vi "Enable Gain Ranging.vi"(0 "session in":T1[](array[typedef]) {"rx baseband session"."3630 session"."Address Space" items=["VXI/VME A16"=1, "VXI/VME A24"=2, "VXI/VME A32"=3, "VXI/VME A64"=4, "PXI Memory Allocations"=9, "PXI Configuration"=10, "PXI BAR0"=11, "PXI BAR1"=12, "PXI BAR2"=13, "PXI BAR3"=14, "PXI BAR4"=15, "PXI BAR5"=16]; "tx baseband session"."3610 session"."Address Space" items=["VXI/VME A16"=1, "VXI/VME A24"=2, "VXI/VME A32"=3, "VXI/VME A64"=4, "PXI Memory Allocations"=9, "PXI Configuration"=10, "PXI BAR0"=11, "PXI BAR1"=12, "PXI BAR2"=13, "PXI BAR3"=14, "PXI BAR4"=15, "PXI BAR5"=16]}, 1 "scope":string(combo), 5 "enable":bool=TRUE, 7 "TRx LO auto-muting":bool=TRUE, 11 "error in":errorcluster) -> (4 "session out":T1[](array[typedef]) {"rx baseband session"."3630 session"."Address Space" items=["VXI/VME A16"=1, "VXI/VME A24"=2, "VXI/VME A32"=3, "VXI/VME A64"=4, "PXI Memory Allocations"=9, "PXI Configuration"=10, "PXI BAR0"=11, "PXI BAR1"=12, "PXI BAR2"=13, "PXI BAR3"=14, "PXI BAR4"=15, "PXI BAR5"=16]; "tx baseband session"."3610 session"."Address Space" items=["VXI/VME A16"=1, "VXI/VME A24"=2, "VXI/VME A32"=3, "VXI/VME A64"=4, "PXI Memory Allocations"=9, "PXI Configuration"=10, "PXI BAR0"=11, "PXI BAR1"=12, "PXI BAR2"=13, "PXI BAR3"=14, "PXI BAR4"=15, "PXI BAR5"=16]}, 15 "error out":errorcluster)   [LabVIEW 2019]
uses:
  TypeDefs/Session.ctl
  <instrlib>/niMmWave/ni3620/Config/v1/Host/Public/High-Level/niMmWave Session.ctl
  <instrlib>/_niInstr/Register Bus/v0/Host/Public/Register Bus Session.ctl
  <instrlib>/_niInstr/Register Bus/v0/Host/Private/Session Data.ctl
  <instrlib>/niMmWave/ni3620/Config/v1/Host/Public/Typedefs/Board Information.ctl
  <instrlib>/niMmWave/ni3620/Config/v1/Host/Public/Typedefs/Hardware Revision.ctl
  <instrlib>/niMmWave/ni3620/Config/v1/Host/Public/Typedefs/Gain Mapping.ctl
  <instrlib>/niMmWave/ni3620/Config/v1/Host/Public/Typedefs/Correction Data.ctl
  <instrlib>/niMmWave/ni3620/Config/v1/Host/Public/Typedefs/Opera Characterization.ctl
  <instrlib>/niMmWave/ni3620/Config/v1/Host/Public/Corrections/Typedefs/Opera Characterization Main Header.ctl
  <instrlib>/niMmWave/ni3620/Config/v1/Host/Public/Corrections/Typedefs/Opera IF Board Information.ctl
  <instrlib>/niMmWave/ni3620/Config/v1/Host/Public/Corrections/Typedefs/Opera Characterization Instance Header.ctl
  <instrlib>/niMmWave/ni3620/Config/v1/Host/Public/Corrections/Typedefs/Opera Characterization Device Data Header.ctl
  <instrlib>/niMmWave/ni3620/Config/v1/Host/Public/Corrections/Typedefs/Opera LO Characterization Data Header.ctl
  <instrlib>/niMmWave/ni3620/Config/v1/Host/Public/Corrections/Typedefs/Opera IF Board Characterization Data Header.ctl
  <instrlib>/niMmWave/ni3620/Config/v1/Host/Public/Corrections/Typedefs/Opera Characterization Device Data.ctl
  <instrlib>/niMmWave/ni3620/Config/v1/Host/Public/Corrections/Typedefs/Opera LO2 Board Characterization Data.ctl
  <instrlib>/niMmWave/ni3620/Config/v1/Host/Public/Corrections/Typedefs/Opera LO Characterization Data.ctl
  <instrlib>/niMmWave/ni3620/Config/v1/Host/Public/Corrections/Typedefs/Opera IF Board Characterization Data.ctl
  <instrlib>/niMmWave/ni3620/Config/v1/Host/Public/Corrections/Typedefs/Opera IQ Impairment Data.ctl
  <instrlib>/niMmWave/ni3620/Config/v1/Host/Public/Typedefs/mmWave Adapter Session Data.ctl
  <instrlib>/niMmWave/ni3620/Config/v1/Host/Public/Typedefs/mmWave Adapter Data.ctl
  <instrlib>/niMmWave/ni3620/Config/v1/Host/Public/Typedefs/mmWave Adapter 2.ctl
  <instrlib>/niMmWave/ni3620/Config/v1/Shared/Typedefs/Subsystem ID.ctl
  <instrlib>/niMmWave/ni3620/Config/v1/Host/Public/Typedefs/mmWave Adapter Channel Information.ctl
  <instrlib>/niMmWave/ni3620/Config/v1/Host/Public/Typedefs/Temperature Coefficients.ctl
  <instrlib>/niMmWave/ni3620/Config/v1/Host/Public/Typedefs/mmWave Characterization.ctl
  <instrlib>/niMmWave/ni3620/Config/v1/Host/Public/Corrections/Typedefs/mmWave Characterization Main Header.ctl
  <instrlib>/niMmWave/ni3620/Config/v1/Host/Public/Corrections/Typedefs/mmWave Characterization Instance Header.ctl
  <instrlib>/niMmWave/ni3620/Config/v1/Host/Public/Typedefs/Session Cache.ctl
  <instrlib>/niMmWave/ni3620/Config/v1/Host/Public/Typedefs/LO2 settings cache.ctl
  <instrlib>/niMmWave/ni3620/Config/v1/Host/Public/Typedefs/LO2 source.ctl
  <instrlib>/niMmWave/ni3620/Config/v1/Host/Public/Typedefs/Desired and Coerced.ctl
  <instrlib>/niMmWave/ni3620/Config/v1/Host/Public/Typedefs/Export cache.ctl
  <instrlib>/niMmWave/ni3620/Config/v1/Host/Public/Typedefs/Path cache.ctl
  <instrlib>/niMmWave/ni3620/Config/v1/Host/Public/Typedefs/Daughterboard Type.ctl
  <instrlib>/niMmWave/ni3620/Config/v1/Host/Public/Typedefs/LO1 settings cache.ctl
  <instrlib>/niMmWave/ni3620/Config/v1/Host/Public/Typedefs/LO1 Source.ctl
  <instrlib>/niMmWave/ni3620/Config/v1/Host/Public/Typedefs/mmWave export cache.ctl
  <instrlib>/niMmWave/ni3620/Config/v1/Host/Private/Board/LO2/LO2 Board Configuration Cache.ctl
  <instrlib>/niMmWave/ni3620/Config/v1/Host/Public/Typedefs/reference clock routing settings.ctl
  <instrlib>/niMmWave/ni3620/Config/v1/Host/Public/Typedefs/LO2 routing settings.ctl
  <instrlib>/niMmWave/ni3620/Config/v1/Host/Private/Board/LO1/LO1 Board Configuration Cache.ctl
  <instrlib>/niMmWave/ni3620/Config/v1/Host/Public/Typedefs/LO1 source settings.ctl
  <instrlib>/niMmWave/ni3620/Config/v1/Host/Public/Typedefs/LO1 export settings.ctl
  <instrlib>/niMmWave/ni3620/Config/v1/Host/Public/Typedefs/LO1 mmWave settings.ctl
  TypeDefs/Tx Baseband Session.ctl
  <instrlib>/niMmWave/ni3610 and ni3630/controls/public/Main Settings.ctl
  <vilib>/Instr/_visa.llb/VISA Register Access Address Space.ctl
  <instrlib>/niMmWave/ni3610 and ni3630/controls/public/Register Adresses.ctl
  <instrlib>/niMmWave/ni3610 and ni3630/controls/public/Base Card Type.ctl
  <instrlib>/niMmWave/ni3610 and ni3630/controls/private/IQ Card Revision.ctl
  <instrlib>/niMmWave/ni3610 and ni3630/controls/public/Board Capability.ctl
  TypeDefs/Blank FPGA Reference.ctl
  TypeDefs/Rx Baseband Session.ctl
  TypeDefs/Hardware Configuration.ctl
  TypeDefs/Direction.ctl
  TypeDefs/Gain Ranging.ctl
  TypeDefs/PXI Trigger Bus Info.ctl
  TypeDefs/Gain Ranging Reference.ctl
  <vilib>/rvi/errors/niLvFpgaAdjustHostInterfaceError.vi
  <vilib>/FPGAPlugInAG/Dynamic/niLvFpga_P2PGetEndpoint_Dynamic.vi
  <vilib>/rvi/interface/nirviReadWriteControl/nirviReadWriteControl.xnode
  <vilib>/rvi/interface/nirviMethod/nirviMethod.xnode
  <instrlib>/niMmWave/ni3620/Config/v1/Host/niMmWave Config v1 Host.lvlib
  <vilib>/rvi/interface/Simulation/niFpgaSimulationCallBeginRW.vi
  NiFpgaLv.dll
  <vilib>/rvi/errors/niLvFpgaMergeErrorWithErrorCode.vi
  <instrlib>/_niInstr/Register Bus/v0/Host/niInstr Register Bus v0 Host.lvlib
  <instrlib>/niMmWave/ni3610 and ni3630/ni3610_and_ni3630_Driver_Lib.lvlib
  <instrlib>/niMmWave/ni3620/Config/v1/Shared/niMmWave Config v1 Shared.lvlib
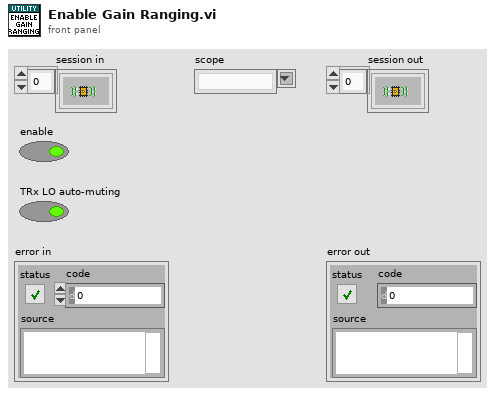
[diagram p1: front panel]
types:
  T1 = typedef "Session.ctl" = cluster{"3620 session":refnum<queue>, "tx baseband session":T2, "rx baseband session":T10, "tx gain (dB)":dbl, "rx gain (dB)":dbl, "hardware configuration":T11, "gain ranging":T13[], "pxi trigger bus information":T14}
  T2 = typedef "Tx Baseband Session.ctl" = cluster{"3610 session":T3, "7902 reference":T9}
  T3 = typedef "ni3610_and_ni3630_Driver_Lib.lvlib/Main Settings.ctl" = cluster{"VISA resource name":refnum<visa-resource-name>, "Address Space":T4, "window_offset":u32, "register_addresses":T5, "required_MM_fpga_version":cluster{"signature":u32, "hardware":u32, "current revision":u32, "oldest revision":u32}, "CPLD Oldest Compat Version ":cluster{"hardware":u32, "CPLD firmware":u32}, "MM_FPGA_image_location":string, "is_init":bool, "card_type":T6, "DacLmkConfigFileName":string, "AdcLmkConfigFileName":string, "AdcConfigFileName":string, "DacConfigFileName_RevA":string, "DacConfigFileName_RevB":string, "Mulde hardware revision":u8, "bypass DAC PLL\n":bool, "IQ Card Revision":T7, "board capability":T8}
  T4 = typedef "VISA Register Access Address Space.ctl" = u16
  T5 = typedef "ni3610_and_ni3630_Driver_Lib.lvlib/Register Adresses.ctl" = cluster{"MM based Registers":cluster{"Revision":u32, "OldestCompatRev":u32, "signature":u32, "scratch":u32, "LedControl":u32, "BoardHwRev":u32, "BoardControl":u32, "ThermalStatus":u32, "BasebandStatus":u32, "BasebandControl":u32, "BasebandAuxSetup":u32, "BasebandAuxStatus":u32, "LmkSyncOutSetup":u32, " AdcSyncOutSetup":u32, " InjSyncOutSetup":u32, " PxiTrig0OutSetup":u32, " PxiTrig1OutSetup":u32, " PxiTrig2OutSetup":u32, " PxiTrig3OutSetup":u32, " PxiTrig4OutSetup":u32, " PxiTrig5OutSetup":u32, " PxiTrig6OutSetup":u32, " PxiTrig7OutSetup":u32}, "CPLD based Registers":cluster{"SlaveSignature":u32, "SlaveRevision":u32, "SlaveOldestCompatRev":u32, "SlaveScratch":u32, "SlaveSetup":u32, "SlaveStatus":u32, "IDacReg_offset":u32, "LMKRegGrp0_offset":u32, "QDacReg_offset":u32, "BrdTempSensorVal":u32, "TempSensorPowerDown":u32, "GPIOReg_offset":u32, "IAdcReg_offset":u32, "QAdcReg_offset":u32, "LMKRegGrp1_offset":u32, "QadcTempSensorVal":u32, "IadcTempSensorVal":u32, "RevisionReg":u32, "VcxoReg":u32, "CpldStatusReg":u32, "PowerReg":u32, "VBiasEnReg":u32, "ExtRefOeReg":u32, "QdacCtrlReg":u32, "QdacStatusReg":u32, "IdacCtrlReg":u32, "IdacStatusReg":u32, "QdacJtagIn":u32, "QdacJtagOut":u32, "IdacJtagIn":u32, "IdacJtagOut":u32, "IqDcSetupReg":u32, "QadcStatusReg":u32, "IadcStatusReg":u32, "BrdSetupReg":u32, "IqDcRevisionReg":u32, "PllStatusReg":u32, "EndpointScratchReg":u32, "AdcSyncCfgReg":u32, "IqCardOpampReg":u32}, "CPLD Register Offset":u32, "MM  Register Offset":u32, " PxiTrig0OutSetup":u32}
  T6 = typedef "ni3610_and_ni3630_Driver_Lib.lvlib/Base Card Type.ctl" = enum16{"unspecified", "ADC", "DAC"}
  T7 = typedef "ni3610_and_ni3630_Driver_Lib.lvlib/IQ Card Revision.ctl" = enum16{"RevA", "RevB", "RevC", "RevD"}
  T8 = typedef "ni3610_and_ni3630_Driver_Lib.lvlib/Board Capability.ctl" = cluster{"baseband sync":enum16{"no baseband sync", "baseband sync"}}
  T9 = typedef "Blank FPGA Reference.ctl" = refnum<k20>
  T10 = typedef "Rx Baseband Session.ctl" = cluster{"3630 session":T3, "7902 reference":T9}
  T11 = typedef "Hardware Configuration.ctl" = cluster{"direction":T12, "baseband only":bool}
  T12 = typedef "Direction.ctl" = enum16{"Transceiver", "Receiver", "Transmitter"}
  T13 = typedef "Gain Ranging.ctl" = cluster{"gain ranging active scope":string, "gain ranging stream session":refnum<k20>}
  T14 = typedef "PXI Trigger Bus Info.ctl" = cluster{"chassis resource name":refnum<visa-resource-name>, "7902R (TX)":i16, "3610 (TX)":i16, "3620 (IF)":i16, "3630 (RX)":i16, "7902R (RX)":i16}
  T15 = typedef "Gain Ranging Reference.ctl" = refnum<k20>
  T16 = cluster{"shift step":i16, "base gain":fxp<+/-,16,12>}
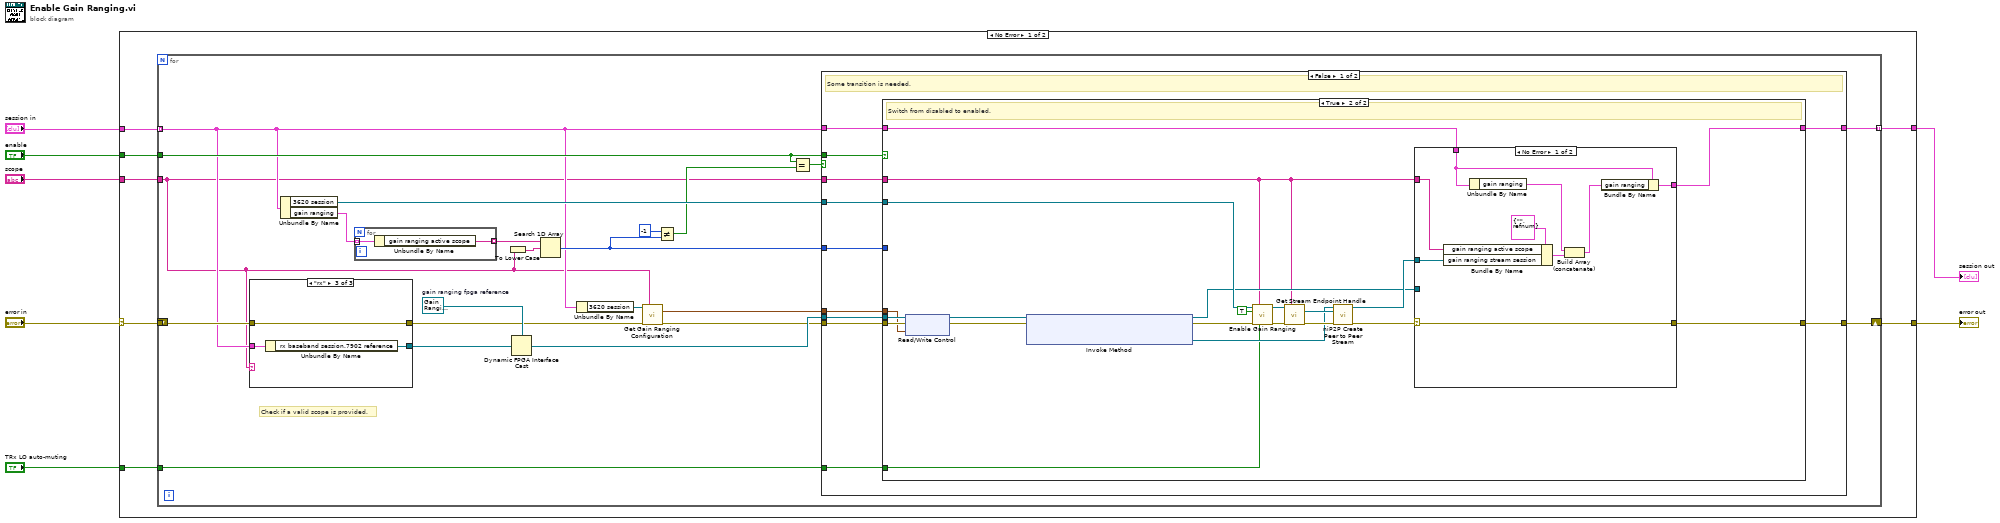
[diagram p0: block diagram]
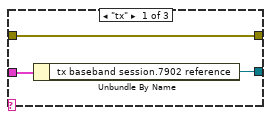
[diagram p2: hidden frame]
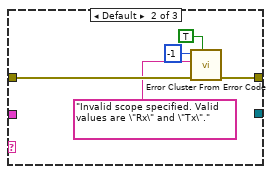
[diagram p3: hidden frame]
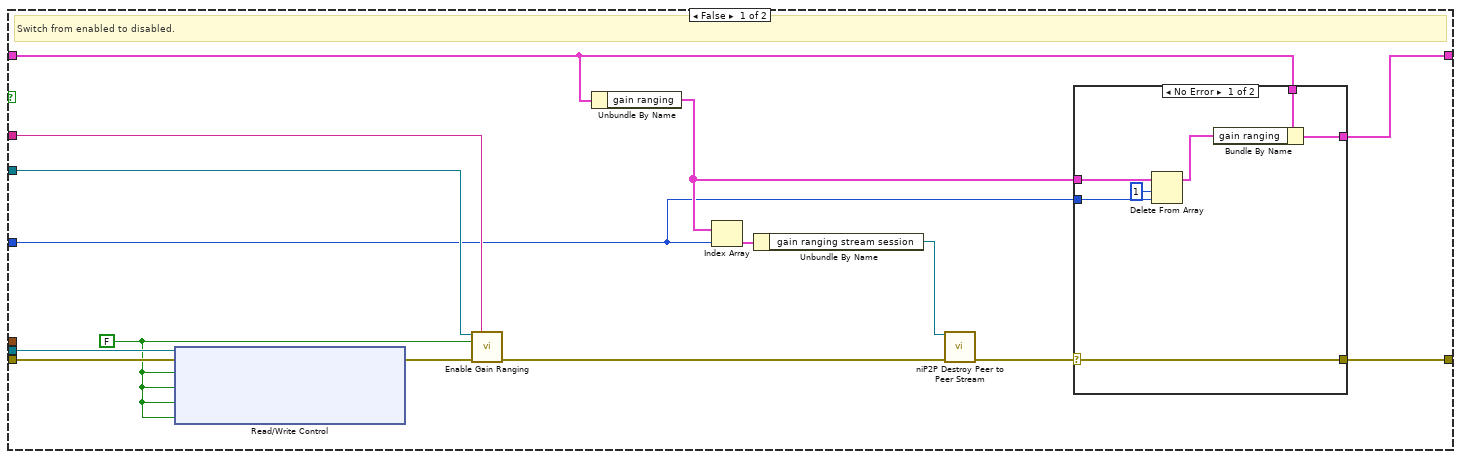
[diagram p4: hidden frame]
diagram:
  n1 = case shown="No Error" "error in" {
    selector: "error in" -> [w9 w120]
    tunnel: [w13 w120] -> w7
    tunnel: "session in" -> [w12 w119]
    tunnel: "enable" -> [w14 _]
    tunnel: "scope" -> [w11 _]
    tunnel: [w10 w119] -> w3
    tunnel: "TRx LO auto-muting" -> [w8 _]
    frame No Error {
      n2 = for {
        tunnel: w14 -> [w30]
        shift-right: [w35] -> w13
        shift-left: w9 -> [w29]
        tunnel: w12 -> [w20] mode=indexing
        tunnel: w11 -> [w19]
        tunnel: [w31] -> w10 mode=indexing
        tunnel: w9 -> [_]
        tunnel: w8 -> [w15]
        w34 = T15 refnum  # gain ranging fpga reference
        # "Check if a valid scope is provided."
        n3 = case shown="\"rx\"" w19 {
          tunnel: [w39 w45 w49] -> w17
          tunnel: w29 -> [w39 w46 w49]
          tunnel: w20 -> [w41 _ w48]
          tunnel: [w40 _ w47] -> w33
          frame "tx" {
            n4 = Unbundle By Name(w41) -> ("tx baseband session.7902 reference"=w40:T9)
          }
          frame Default {
            n5 = call <vilib>:"Error Cluster From Error Code.vi"("show call chain? (False)"=TRUE, "error in (no error)"=w46, "error message (\"\")"="Invalid scope specified. Valid values are \"Rx\" and \"Tx\"." ("error message (\"\")"), "error code (0)"=-1) -> ("error out"=w45:errorcluster)  [unwired: 5 in]
          }
          frame "rx" {
            n6 = Unbundle By Name(w48) -> ("rx baseband session.7902 reference"=w47:T9)
          }
        }
        n7 = Unbundle By Name(w20) -> ("3620 session"=w32:refnum<queue>, "gain ranging"=w26:T13[])
        n8 = for {
          tunnel: w26 -> [w38] mode=indexing
          tunnel: [w37] -> w28 mode=indexing
          n9 = Unbundle By Name(w38) -> ("gain ranging active scope"=w37:string)
        }
        n10 = To Lower Case(string=w19) -> (all lower case string=w27:string)
        n11 = Dynamic FPGA Interface Cast(Session In=w34, Type=w33) -> (Session Out=w36:T15)
        n12 = Search 1D Array(1D array=w28, element=w27) -> (index of element=w22:i32)  [unwired: 1 in]
        n13 = Unbundle By Name(w20) -> ("3620 session"=w21:refnum<queue>)
        n14 = call <instrlib>:"Get Gain Ranging Configuration.vi"("session in"=w21, "scope"=w19, "error in"=w17) -> ("table info"=w18:T16, "error out"=w16:errorcluster)  [unwired: 10 in, 1 out]
        n15 = Not Equal?(x=-1, y=w22) -> (x != y?=w24:bool)
        n16 = Equal?(x=w30, y=w24) -> (x = y?=w23:bool)
        n17 = case shown="False" w23 {
          tunnel: w20 -> [w60 w117]
          tunnel: w36 -> [w59 _]
          tunnel: [w58 w118] -> w35
          tunnel: w16 -> [w57 w118]
          tunnel: w32 -> [w56 _]
          tunnel: [w55 w117] -> w31
          tunnel: w19 -> [w54 _]
          tunnel: w30 -> [w53 _]
          tunnel: w22 -> [w52 _]
          tunnel: w18 -> [w51 _]
          tunnel: w15 -> [w50 _]
          frame False {
            # "Some transition is needed."
            n18 = case shown="True" w53 {
              tunnel: w57 -> [w75 w102]
              tunnel: [w67 w94] -> w58
              tunnel: w59 -> [w74 w101]
              tunnel: w56 -> [w72 w103]
              tunnel: w54 -> [w68 w86]
              tunnel: w60 -> [w70 w97]
              tunnel: [w69 w95] -> w55
              tunnel: w52 -> [w62 _]
              tunnel: w51 -> [_ w89]
              tunnel: w50 -> [_ w85]
              frame False {
                w61 = FALSE ("gain ranging.enable")
                # "Switch from enabled to disabled."
                n19 = xnode "Read/Write Control"("FPGA VI Reference In"=w74, "error in"=w75, "gain ranging.enable"=w61, "gain ranging.enable fine gain ranging"=w61, "gain ranging.enable coarse gain ranging"=w61, "gain ranging.enable port config"=w61) -> ("error out"=w73:errorcluster)  [unwired: 1 out]
                n20 = call <instrlib>:"Enable Gain Ranging.vi"("session in"=w72, "scope"=w68, "enable gain ranging?"=w61, "error in"=w73) -> ("error out"=w71:errorcluster)  [unwired: 10 in, 1 out]
                n21 = Unbundle By Name(w70) -> ("gain ranging"=w63:T13[])
                n22 = Index Array(array=w63, index=w62) -> (element=w65:T13)
                n23 = Unbundle By Name(w65) -> ("gain ranging stream session"=w64:refnum<k20>)
                n24 = call <vilib>:"niP2P Destroy Peer to Peer Stream.vi"("stream session"=w64, "error in (no error)"=w71) -> ("error out"=w66:errorcluster)  [unwired: 13 in]
                n25 = case shown="No Error" w66 {
                  selector: w66 -> [w80 w83]
                  tunnel: w70 -> [w82 w84]
                  tunnel: [w81 w84] -> w69
                  tunnel: [w80 w83] -> w67
                  tunnel: w63 -> [w79 _]
                  tunnel: w62 -> [w78 _]
                  frame No Error {
                    n26 = Delete From Array(array=w79, length=1, index=w78) -> (array with subset deleted=w76:T13[])  [unwired: 1 out]
                    n27 = Bundle By Name(cluster=w82, "gain ranging"=w76) -> (w81:T1)
                  }
                  frame Error {
                  }
                }
              }
              frame True {
                # "Switch from disabled to enabled."
                n28 = xnode "Read/Write Control"("FPGA VI Reference In"=w101, "error in"=w102, "table info"=w89) -> ("FPGA VI Reference Out"=w91:T15, "error out"=w90:errorcluster)
                n29 = xnode "Invoke Method"("FPGA VI Reference In"=w91, "error in"=w90) -> ("FPGA VI Reference Out"=w92:T15, "error out"=w100:errorcluster, "Writer"=w99:refnum<k20>)
                n30 = call <instrlib>:"Enable Gain Ranging.vi"("session in"=w103, "scope"=w86, "enable gain ranging?"=TRUE, "error in"=w100, "TRx LO auto-muting"=w85) -> ("session out"=w88:refnum<queue>, "error out"=w87:errorcluster)  [unwired: 9 in]
                n31 = call <instrlib>:"Get Stream Endpoint Handle.vi"("session in"=w88, "scope"=w86, "error in"=w87) -> ("reader handle"=w105:refnum<k20>, "error out"=w104:errorcluster)  [unwired: 10 in, 1 out]
                n32 = call <vilib>:"niP2P Create Peer to Peer Stream.vi"("writer"=w99, "reader"=w105, "error in (no error)"=w104) -> ("stream session"=w96:refnum<k20>, "error out"=w93:errorcluster)  [unwired: 11 in]
                n33 = case shown="No Error" w93 {
                  selector: w93 -> [w114 w115]
                  tunnel: w97 -> [w110 w116]
                  tunnel: w96 -> [w111 _]
                  tunnel: w86 -> [w112 _]
                  tunnel: [w109 w116] -> w95
                  tunnel: [w114 w115] -> w94
                  tunnel: w92 -> [_ _]
                  frame No Error {
                    n34 = Bundle By Name(cluster=T13 {"gain ranging active scope"="", "gain ranging stream session"=refnum} ("gain ranging"), "gain ranging active scope"=w112, "gain ranging stream session"=w111) -> (w108:T13)
                    n35 = Unbundle By Name(w110) -> ("gain ranging"=w107:T13[])
                    n36 = Build Array (concatenate)(w107, w108) -> (w106:T13[])
                    n37 = Bundle By Name(cluster=w110, "gain ranging"=w106) -> (w109:T1)
                  }
                  frame Error {
                  }
                }
              }
            }
          }
          frame True {
            # "No transition is needed.  Do nothing."
          }
        }
      }
    }
    frame Error {
    }
  }
  "error out" <- w7
  "session out" <- w3
